vi "buffer_data.vi"(8 "error in":errorcluster, 10 "data in":T1, 11 "command":T2) -> (0 "error out":errorcluster, 1 "time out?":bool, 2 "data out":T1)   [LabVIEW 2017]
uses:
  Control/buffer_data_command.ctl
  Control/buff_data_type.ctl
panel:
  out "Number of elements in queue":i32 caption="キューの中の要素数"
  # "Number of elements in queue"
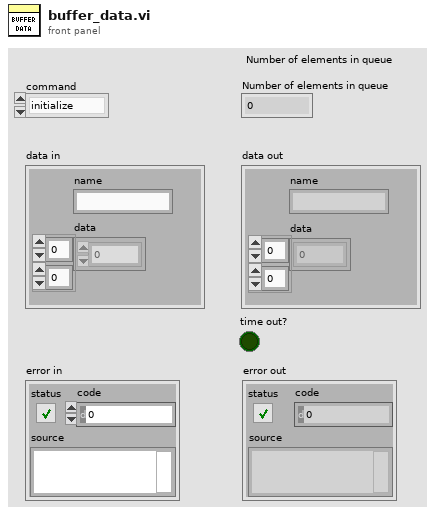
[diagram p1: front panel]
types:
  T1 = typedef "buff_data_type.ctl" = cluster{"name":string, "data":dbl[][]}
  T2 = typedef "buffer_data_command.ctl" = enum16{"initialize", "Enqueue", "Dequeue", "end"}
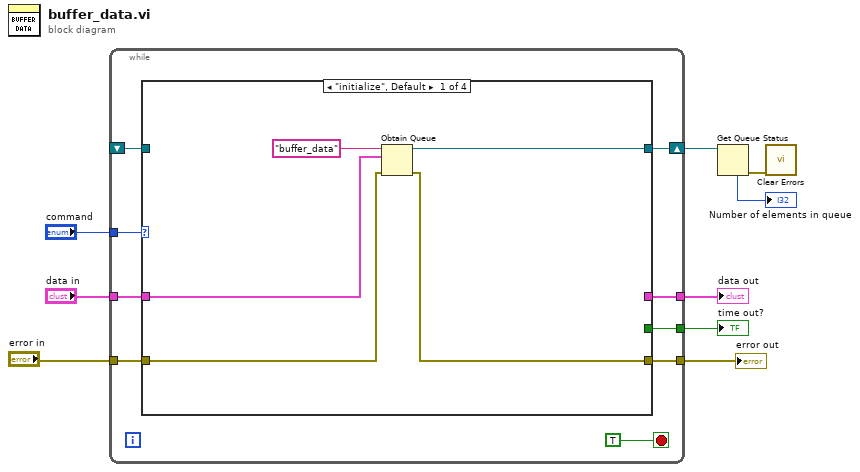
[diagram p0: block diagram]
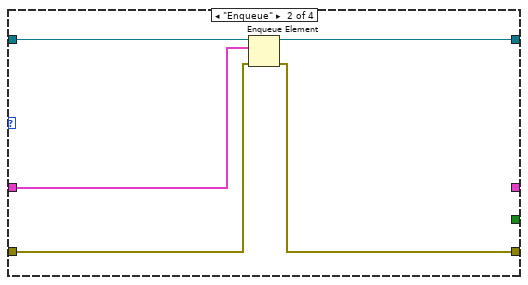
[diagram p2: hidden frame]
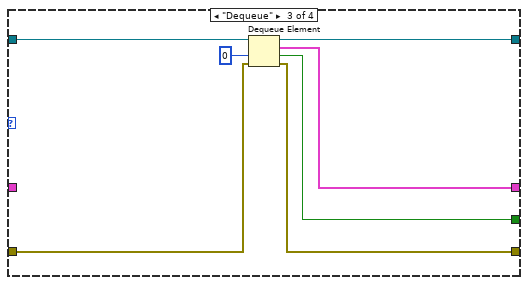
[diagram p3: hidden frame]
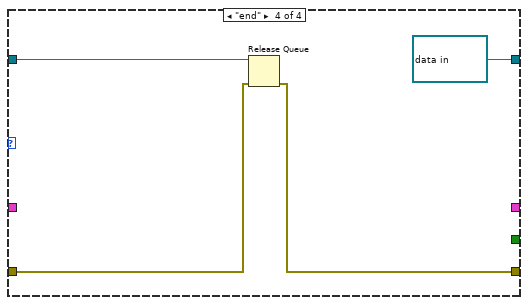
[diagram p4: hidden frame]
diagram:
  n1 = while {
    tunnel: "command" -> [w17]
    tunnel: "data in" -> [w15]
    shift-right: [w16] -> w5
    shift-left: _ -> [w14]
    tunnel: [w13] -> w7
    tunnel: "error in" -> [w12]
    tunnel: [w11] -> w1
    tunnel: [w10] -> w6
    stop <- TRUE stop-if-true
    n2 = case shown="\"initialize\", Default" w17 {
      tunnel: [w23 w26 w34 refnum<queue> refnum ("queue out")] -> w16
      tunnel: w15 -> [w21 w27 _ _]
      tunnel: w14 -> [_ w28 w35 w39]
      tunnel: [_ _ w32 _] -> w13
      tunnel: w12 -> [w20 w25 w31 w37]
      tunnel: [w19 w24 w30 w38] -> w11
      tunnel: [_ _ w29 _] -> w10
      frame "initialize", Default {
        n3 = Obtain Queue(name (unnamed)="buffer_data" ("名前（名前なし）"), element data type=w21, error in (no error)=w20) -> (queue out=w23:refnum<queue>, error out=w19:errorcluster)  [unwired: 2 in, 1 out]
      }
      frame "Enqueue" {
        n4 = Enqueue Element(queue=w28, element=w27, error in (no error)=w25) -> (queue out=w26:refnum<queue>, error out=w24:errorcluster)  [unwired: 1 in, 1 out]
      }
      frame "Dequeue" {
        n5 = Dequeue Element(queue=w35, timeout in ms (-1)=0 ("タイムアウト（ms）（-1）"), error in (no error)=w31) -> (queue out=w34:refnum<queue>, element=w32:T1, timed out?=w29:bool, error out=w30:errorcluster)
      }
      frame "end" {
        n6 = Release Queue(queue=w39, error in (no error)=w37) -> (error out=w38:errorcluster)  [unwired: 1 in, 2 out]
      }
    }
  }
  "data out" <- w7
  "time out?" <- w6
  "error out" <- w1
  n7 = Get Queue Status(queue=w5) -> (error out=w3:errorcluster, # elements in queue=→"Number of elements in queue":i32)  [unwired: 2 in, 6 out]
  n8 = call <vilib>:"Clear Errors.vi"("error in (no error)"=w3) -> ()  [unwired: 5 in, 2 out]
